vi "test Error Code.vi"(8 "error in (no error)":errorcluster, 11 "TestCase in":refnum<class "Parameter Setting.lvclass">) -> (0 "error out":errorcluster, 3 "TestCase out":refnum<class "Parameter Setting.lvclass">)   [LabVIEW 2017, in "Deterministic Error Tests.lvlib" / "Parameter Setting.lvclass"]
uses:
  Parameter Setting.lvclass
  Parameter Setting.lvclass/Parameter Setting.ctl
  <vilib>/addons/_JKI Toolkits/VI Tester/TestCase.llb/TestCase.lvclass
  Source/Deterministic Error Builder.lvlib
  C:/Program Files (x86)/National Instruments/LabVIEW 2017/vi.lib/addons/_JKI Toolkits/VI Tester/TestCase.llb/TestCase.lvclass
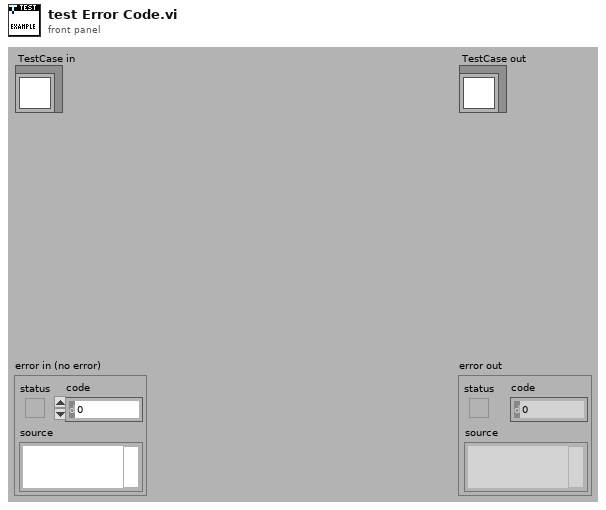
[diagram p1: front panel]
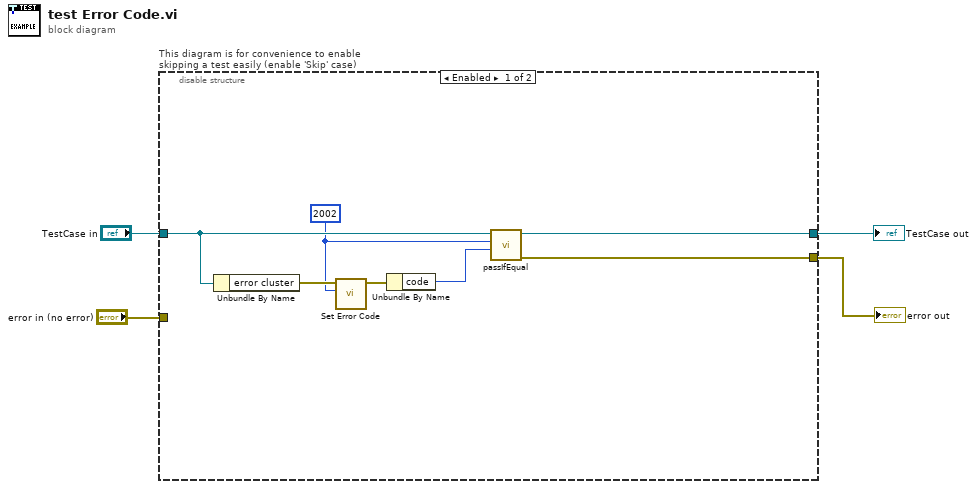
[diagram p0: block diagram]
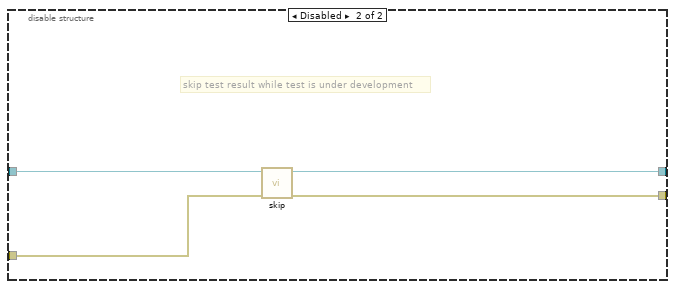
[diagram p2: hidden frame]
diagram:
  n1 = disable-structure "This diagram is for convenience to enable skipping a test easily (enable 'Skip' case)" shown="Enabled" {
    disable-tunnel: "TestCase in" -> [w9 w15]
    disable-tunnel: [w11 w13] -> w2
    disable-tunnel: [w10 w14] -> w1
    disable-tunnel: "error in (no error)" -> [_ w12]
    frame Enabled {
      w5 = 2002 ("code")
      n2 = Unbundle By Name(w9) -> ("error cluster"=w7:errorcluster)
      n3 = call "Set Error Code.vi"("code"=w5, "error in"=w7) -> ("error out"=w6:errorcluster)  [unwired: 9 in]
      n4 = Unbundle By Name(w6) -> ("code"=w8:i32)
      n5 = call-dynamic "passIfEqual.vi"("y"=w8, "x"=w5, "TestCase in"=w9) -> ("error out"=w10:errorcluster, "TestCase out"=w11:refnum<class "Parameter Setting.lvclass">)  [unwired: 7 in]
    }
    frame Disabled {
      # "skip test result while test is under development"
      n6 = call <vilib>:"skip.vi"("error in (no error)"=w12, "TestCase in"=w15) -> ("error out"=w14:errorcluster, "TestCase out"=w13:refnum<class "Parameter Setting.lvclass">)  [unwired: 8 in]
    }
  }
  "error out" <- w1
  "TestCase out" <- w2
